vi "subImage_Pad.vi"(6 "ROI":T1={"Bin"=2, "ROI"={"x offset"=256, "y offset"=256, "x width"=512, "y width"=512}} {"ROI"."x offset" min=0 max=2048 step=1; "ROI"."y offset" min=0 max=2048 step=1; "ROI"."x width" min=0 max=2048 step=1; "ROI"."y width" min=0 max=2048 step=1; "Bin" items=["1x1"=1, "2x2"=2, "4x4"=4]}, 8 "Error In":errorcluster, 11 "Image in":u16[][](graph)=array1024x1024[1048576 elements]) -> (0 "Error out":errorcluster, 1 "Image calculation":u16[][](graph), 3 "Image out":u16[][](graph))   [LabVIEW 2015]
panel:
  # "Pad zeros around the actual image to get the \"full image\" for the given bin size"
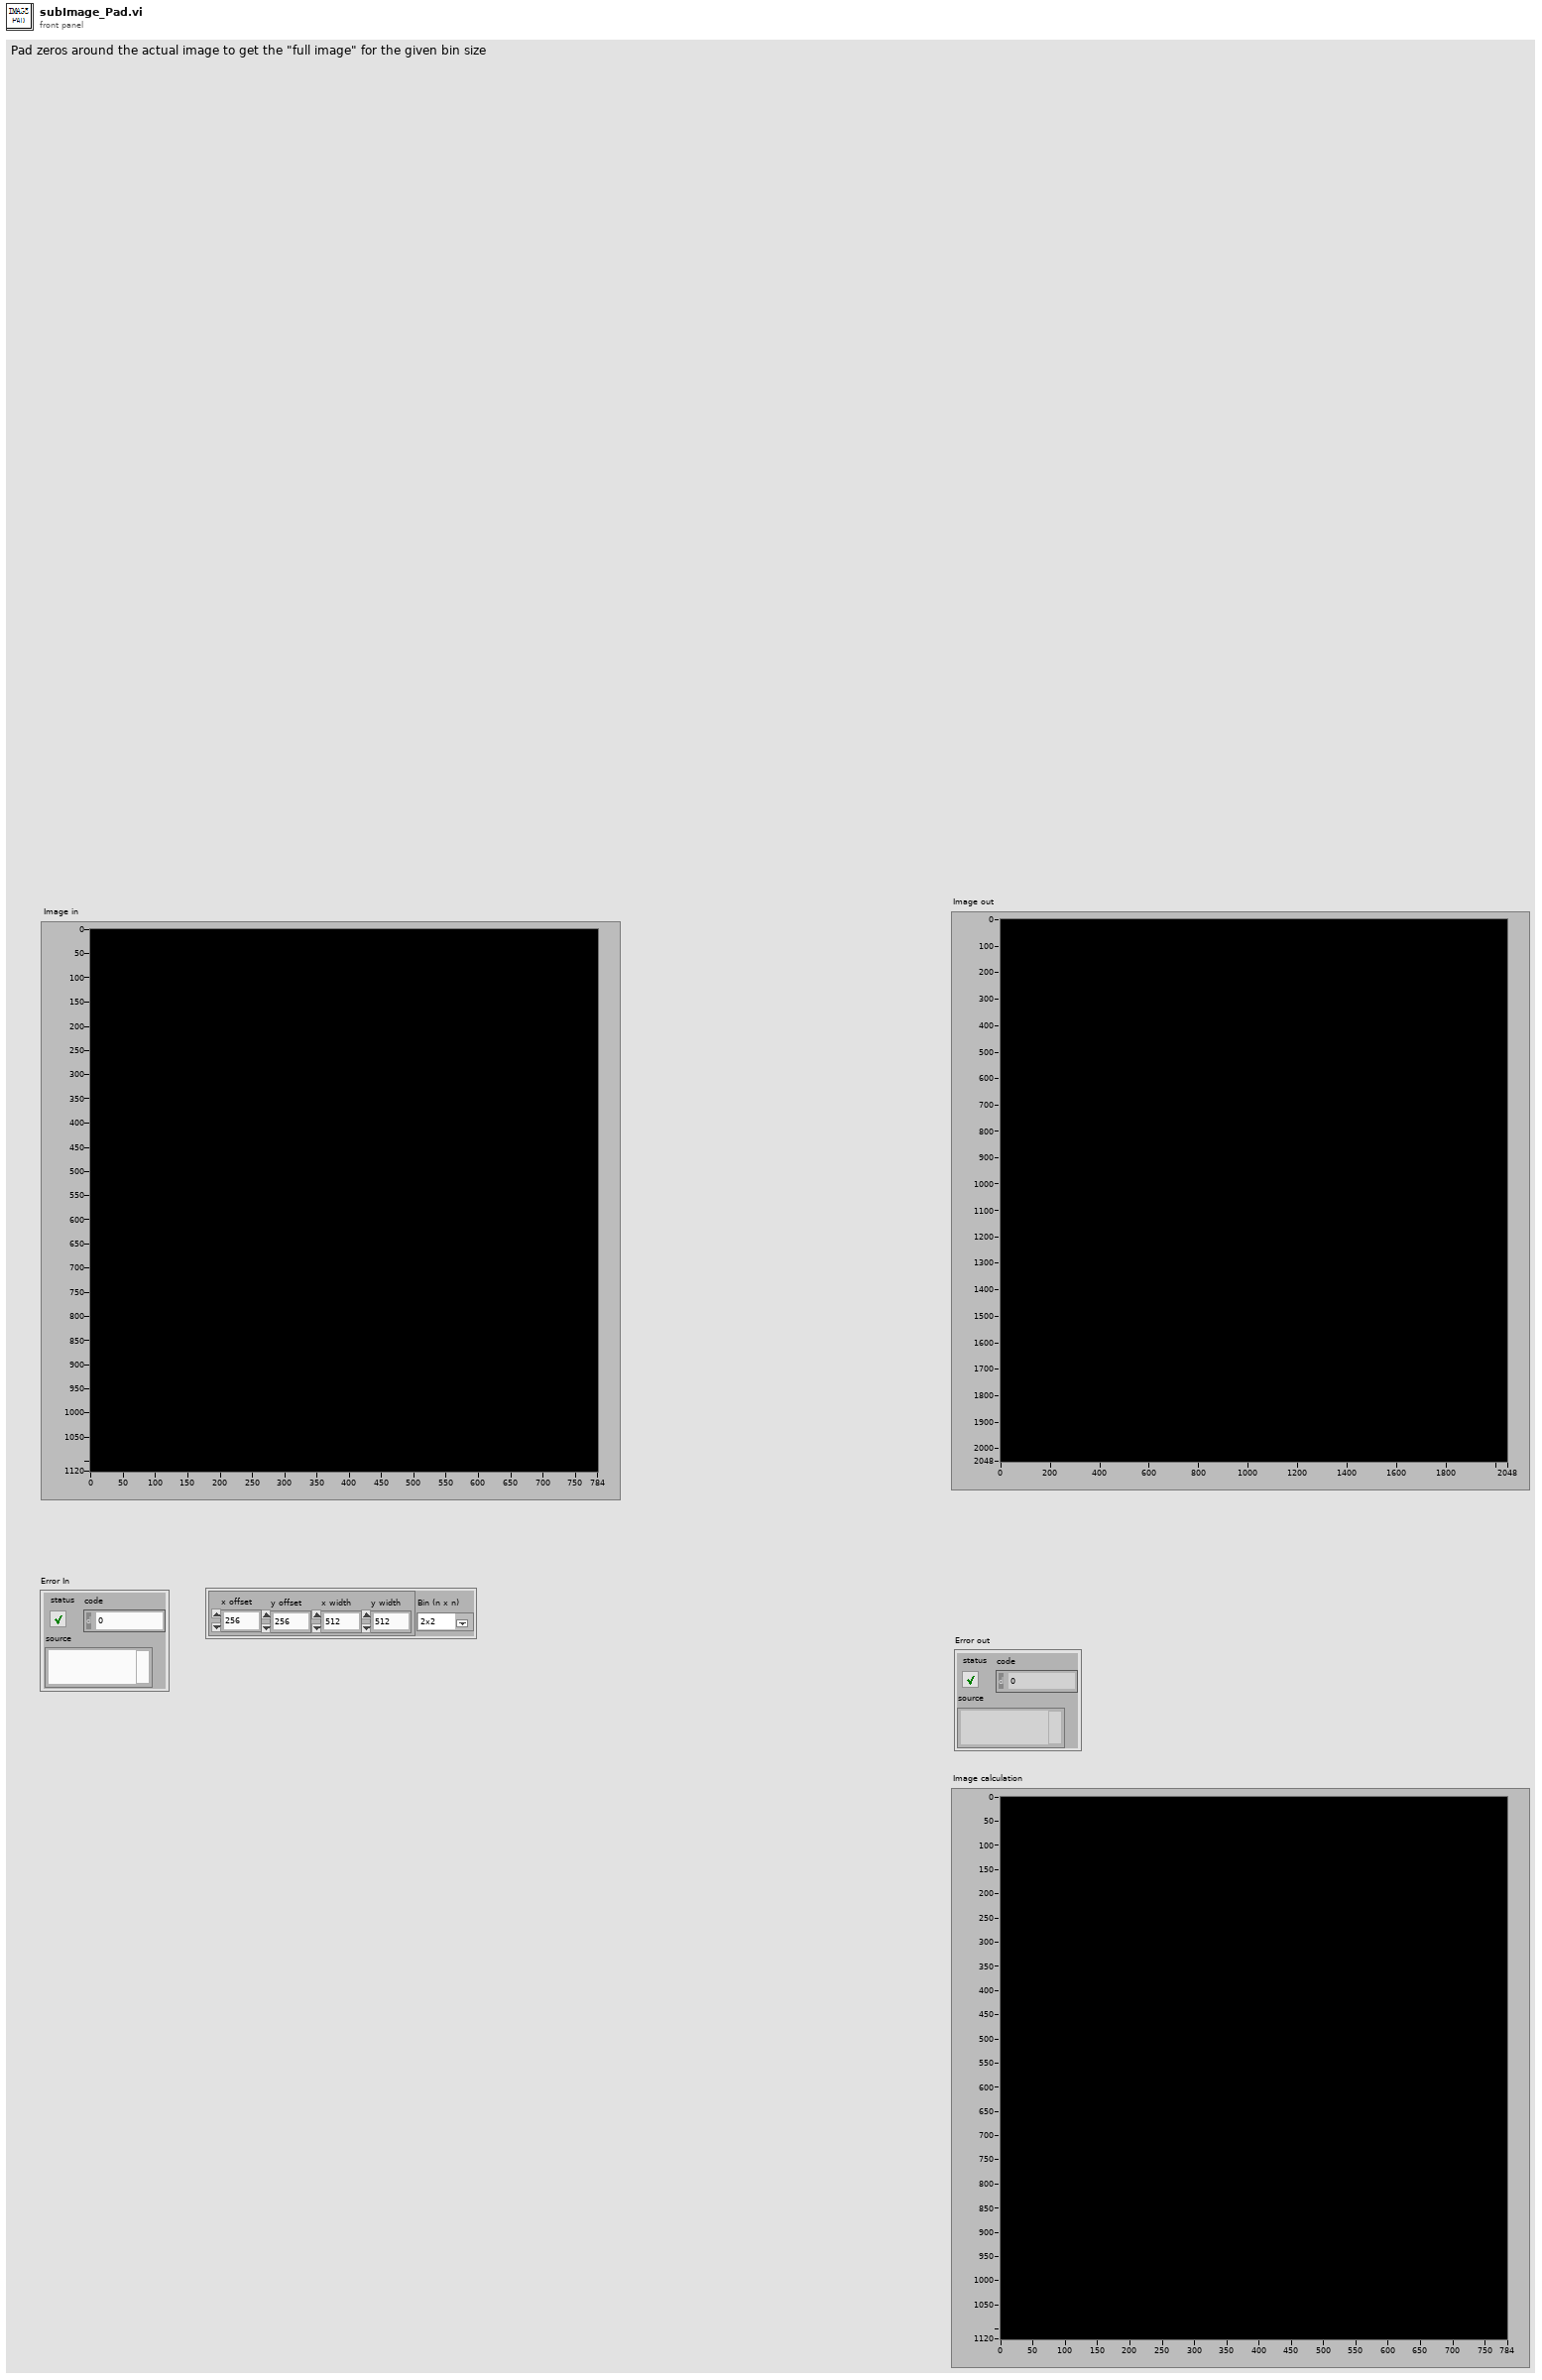
[diagram p1: front panel]
types:
  T1 = cluster{"Bin":u16, "ROI":cluster{"x offset":i32, "y offset":i32, "x width":i32, "y width":i32}}
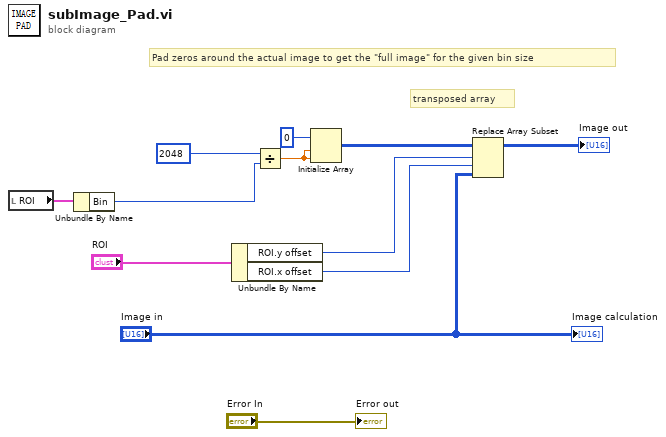
[diagram p0: block diagram]
diagram:
  # "transposed array"
  # "Pad zeros around the actual image to get the \"full image\" for the given bin size"
  n1 = local read "ROI"() -> (w4:T1)
  n2 = Unbundle By Name(w4) -> ("Bin"=w3:u16)
  n3 = Unbundle By Name("ROI") -> ("ROI.y offset"=w7:i32, "ROI.x offset"=w11:i32)
  n4 = Divide(x=u16 2048 ("element"), y=w3) -> (x/y=w9:dbl)
  n5 = Initialize Array(u16 0 ("element"), w9, w9) -> (w2:u16[][])
  n6 = Replace Array Subset(array=w2, new element="Image in", index (row)=w7, index (col)=w11) -> (→"Image out":u16[][])
  "Error out" <- "Error In"
  "Image calculation" <- "Image in"
